vi "Filter 1D Array with Scalar (U16)__ogtk.vi"(5 "items to filter":u16, 6 "array":u16[](array[numeric])) -> (1 "filtered item indices":i32[](array[numeric]), 2 "filtered array":u16[](array[numeric]))   [LabVIEW 2018]
doc: "This polymorphic VI filters out all instances of <B>items to filter</B> from the input <B>array</B> and outputs the result as <B>filtered array</B> along with an array of <B>filtered item indices</B> containing the indices of the items that were filtered. You can wire either a 1D array or a scalar value to <B>items to filter</B>."
uses:
  <userlib>/_OpenG.lib/array/array.llb/Search 1D Array (U16)__ogtk.vi
  <userlib>/_OpenG.lib/array/array.llb/Delete Elements from 1D Array (U16)__ogtk.vi
panel:
  # "Filter 1D Array.vi\n\nFilters items from a source array VIs in memory whose front panels are open.\n\nPlease visit http://www.OpenG.org to learn about the\nOpen Source LabVIEW software movement.\n\nNOTICE -- YOU MUST LEAVE THIS NOTICE IN PLACE.  PER THE TERMS OF THE LICENSE BELOW, YOU MAY SUBLICENSE THIS SOFTWARE \nIN ANY WAY THAT DOES NOT CONFLICT WITH THIS LICENSE.\n\n### BSD License (http://www.opensource.org/licenses/bsd-license.php) Begin ###\n \nCopyright (c) 2002-2006, Jim Kring <jim@jimkring.com>\n\nAll rights reserved.\n\nRedistribution and use in source and binary forms, with or without modification, are permitted provided that the following conditions are met:\n\n    * Redistributions of source code must retain the above copyright notice, this list of conditions and the following disclaimer.\n    * Redistributions in binary form must reproduce the above copyright notice, this list of conditions and the following disclaimer in the \n       documentation and/or other materials provided with the distribution.\n    * Neither the name of SciWare, James Kring, Inc., nor the names of its contributors may be used to endorse or promote products derived \n       from this software without specific prior written permission.\n\nTHIS SOFTWARE IS PROVIDED BY THE COPYRIGHT HOLDERS AND CONTRIBUTORS \"AS IS\" AND ANY EXPRESS OR IMPLIED WARRANTIES, \nINCLUDING, BUT NOT LIMITED TO, THE IMPLIED WARRANTIES OF MERCHANTABILITY AND FITNESS FOR A PARTICULAR PURPOSE ARE \nDISCLAIMED. IN NO EVENT SHALL THE COPYRIGHT OWNER OR CONTRIBUTORS BE LIABLE FOR ANY DIRECT, INDIRECT, INCIDENTAL,\n SPECIAL, EXEMPLARY, OR CONSEQUENTIAL DAMAGES (INCLUDING, BUT NOT LIMITED TO, PROCUREMENT OF SUBSTITUTE GOODS OR \nSERVICES; LOSS OF USE, DATA, OR PROFITS; OR BUSINESS INTERRUPTION) HOWEVER CAUSED AND ON ANY THEORY OF LIABILITY, \nWHETHER IN CONTRACT, STRICT LIABILITY, OR TORT (INCLUDING NEGLIGENCE OR OTHERWISE) ARISING IN ANY WAY OUT OF THE USE \nOF THIS SOFTWARE, EVEN IF ADVISED OF THE POSSIBILITY OF SUCH DAMAGE.\n\n### BSD License End ###"
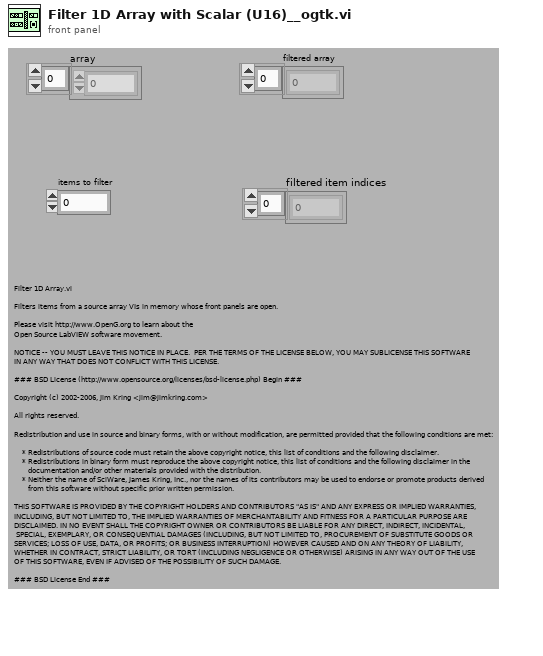
[diagram p1: front panel]
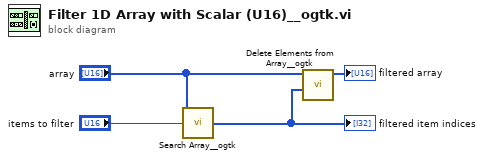
[diagram p0: block diagram]
diagram:
  n1 = call-poly <userlib>:"Search Array__ogtk.vi"("Array"="array", "Element Data"="items to filter") -> ("Indices of Elements"=w1:i32[])  [unwired: 7 in]
  "filtered item indices" <- w1
  n2 = call-poly <userlib>:"Delete Elements from Array__ogtk.vi"("indices"=w1, "array"="array") -> ("array w/ subset deleted"=→"filtered array":u16[])  [unwired: 8 in, 1 out]
